vi "数组数据运算-比较.vi"() -> ()   [LabVIEW 2014]
panel:
  out "结果2":bool
  out "结果1":bool[](array[boolean])
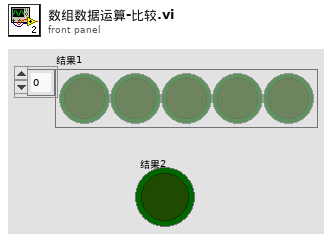
[diagram p1: front panel]
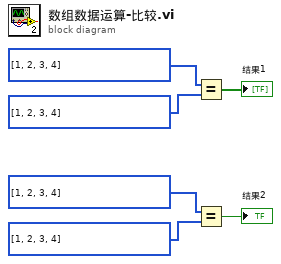
[diagram p0: block diagram]
diagram:
  n1 = Equal?(x=i32[] [1, 2, 3, 4], y=i32[] [1, 2, 3, 4]) -> (x = y?=→"结果1":bool[])
  n2 = Equal?(x=i32[] [1, 2, 3, 4], y=i32[] [1, 2, 3, 4]) -> (x = y?=→"结果2":bool)
